vi "Powermeter_eom.vi"() -> ()   [LabVIEW 2016]
uses:
  <vilib>/userdefined/High Color/nirio_resource_hc.ctl
  <vilib>/FPGAPlugInAG/PXIe-7847R/niLvFpga_Open_PXIe-7847R.vi
  <vilib>/FPGAPlugInAG/PXIe-7847R/niLvFpga_Run_PXIe-7847R.vi
  <vilib>/Utility/error.llb/Error Cluster From Error Code.vi
  <vilib>/rvi/errors/niLvFpgaAdjustHostInterfaceError.vi
  <vilib>/Utility/file.llb/Write Delimited Spreadsheet (DBL).vi
  <vilib>/rvi/interface/nirviOpenFPGA/nirviOpenFPGA.xnode
  LabView Code/FPGA code/FPGA Bitfiles/Microspherefeedb_FPGATarget_MyCompilation_PIDXYZ_eom.lvbitx
  <vilib>/rvi/interface/nirviMethod/nirviMethod.xnode
  <vilib>/rvi/interface/nirviReadWriteControl/nirviReadWriteControl.xnode
  NiFpgaLv.dll
panel:
  in  "RIO Device":T1="RIO0"
  in  "N of steps":i32=401
  in  "step size":dbl=0.05
  in  "Start":dbl=-10.0
  in  "file path (dialog if empty)":path=path "C:/data/20180123/EOM_characterization/meas3.txt"
  out "Array":dbl[][](array[numeric])=[[0.000150393869, -10.0], [0.000149684973, -9.95], [0.000149058935, -9.9], [0.000148333784, -9.85], [0.000147686165, -9.8], [0.000147031693, -9.75], [0.0001463441, -9.7], [0.000145612459, -9.65], [0.000144846243, -9.6], [0.000144049729, -9.55], [0.000143292942, -9.5], [0.00014244036, -9.45], [0.000141621495, -9.4], [0.000140752702, -9.35], [0.000139932832, -9.3], [0.00013900231, -9.25], [0.000138039162, -9.2], [0.000137029376, -9.15], [0.000136068833, -9.1], [0.000135099486, -9.05], [0.000134103757, -9.0], [0.000133110167, -8.95], [0.000132204717, -8.9], [0.000131523033, -8.85], [0.000130512242, -8.8], [0.000129471417, -8.75], [0.000128434986, -8.7], [0.000127368286, -8.65], [0.00012630847, -8.6], [0.000125196137, -8.55], [0.00012410841, -8.5], [0.000123014004, -8.45], [0.000121917823, -8.4], [0.000120789067, -8.35], [0.000119675235, -8.3], [0.000118584379, -8.25], [0.00011747158, -8.2], [0.00011635691, -8.15], [0.00011528789, -8.1], [0.00011419248, -8.05], [0.000113120914, -8.0], [0.000112039837, -7.949999999999999], [0.000110946967, -7.9], [0.000109817694, -7.85], [0.000108703345, -7.8], [0.000107574131, -7.75], [0.000106449981, -7.699999999999999], [0.000105339168, -7.65], [0.000104231709, -7.6], [0.000103070852, -7.55], [0.000101967875, -7.5], [0.000100871737, -7.449999999999999], [9.97827883e-05, -7.4], [9.86708983e-05, -7.35], [9.75727817e-05, -7.3], [9.6466043e-05, -7.25], [9.53593917e-05, -7.199999999999999], [9.42729966e-05, -7.15], [9.31596442e-05, -7.1], [9.20545936e-05, -7.05], [9.0971429e-05, -7.0], [8.98795406e-05, -6.949999999999999], [8.87838905e-05, -6.9], [8.76979248e-05, -6.85], [8.66194823e-05, -6.8], [8.55211401e-05, -6.75], [8.44504029e-05, -6.699999999999999], [8.33811646e-05, -6.65], [8.23208466e-05, -6.6], [8.12596481e-05, -6.55], [8.02040886e-05, -6.5], [7.91571947e-05, -6.449999999999999], [7.80946066e-05, -6.4], [7.70534461e-05, -6.35], [7.60166076e-05, -6.3], [7.49777828e-05, -6.25], [7.39377138e-05, -6.199999999999999], [7.2927709e-05, -6.15], [7.19085219e-05, -6.1], [7.09057058e-05, -6.05], [6.99179145e-05, -6.0], [6.90001907e-05, -5.95], [6.81280071e-05, -5.8999999999999995], [6.72356837e-05, -5.85], [6.63338506e-05, -5.8], [6.53637835e-05, -5.75], [6.44089887e-05, -5.7], [6.34148528e-05, -5.6499999999999995], [6.24612585e-05, -5.6], [6.15193494e-05, -5.55], [6.05423993e-05, -5.5], [5.95535821e-05, -5.45], [5.8533682e-05, -5.3999999999999995], [5.7534915e-05, -5.35], [5.65688533e-05, -5.3], [5.5614415e-05, -5.25], [5.46966367e-05, -5.199999999999999], [5.37870292e-05, -5.1499999999999995], [5.28832607e-05, -5.1], [5.19945861e-05, -5.05], [5.11113103e-05, -5.0], [5.02308103e-05, -4.949999999999999], [4.93651132e-05, -4.8999999999999995], [4.85076816e-05, -4.85], [4.7653044e-05, -4.8], [4.6811776e-05, -4.75], [4.59838811e-05, -4.699999999999999], [4.51689448e-05, -4.6499999999999995], [4.43613535e-05, -4.6], [4.35506627e-05, -4.55], [4.27679734e-05, -4.5], [4.20016877e-05, -4.449999999999999], [4.12174413e-05, -4.3999999999999995], [4.04428574e-05, -4.35], [3.96582109e-05, -4.3], [3.88736553e-05, -4.25], [3.81013197e-05, -4.199999999999999], [3.73277762e-05, -4.1499999999999995], [3.65616252e-05, -4.1], [3.58079087e-05, -4.05], [3.50554728e-05, -4.0], [3.43142165e-05, -3.9499999999999993], [3.35744189e-05, -3.8999999999999995], [3.28419919e-05, -3.8499999999999996], [3.21193183e-05, -3.8], [3.14002464e-05, -3.75], [3.06878501e-05, -3.6999999999999993], [2.99921649e-05, -3.6499999999999995], [2.92990935e-05, -3.5999999999999996], [2.86223167e-05, -3.55], [2.79571123e-05, -3.5], [2.72917787e-05, -3.4499999999999993], [2.66343632e-05, -3.3999999999999995], [2.59851477e-05, -3.3499999999999996], [2.53385915e-05, -3.3], [2.46998134e-05, -3.25], [2.40559821e-05, -3.1999999999999993], [2.34006638e-05, -3.1499999999999995], [2.27987748e-05, -3.0999999999999996], [2.21989449e-05, -3.05], [2.1609243e-05, -3.0], [2.10390936e-05, -2.9499999999999993], [2.04805674e-05, -2.8999999999999995], [1.99267452e-05, -2.8499999999999996], [1.93897922e-05, -2.8], [1.8847466e-05, -2.75], [1.83229949e-05, -2.6999999999999993], [1.78147784e-05, -2.6499999999999995], [1.73084863e-05, -2.5999999999999996], [1.68125953e-05, -2.55], [1.63255063e-05, -2.5], [1.58559433e-05, -2.4499999999999993], [1.53885012e-05, -2.3999999999999995], [1.49266416e-05, -2.3499999999999996], [1.44811456e-05, -2.3], [1.40492502e-05, -2.25], [1.36235085e-05, -2.1999999999999993], [1.32113801e-05, -2.1499999999999995], [1.28091506e-05, -2.0999999999999996], [1.24163826e-05, -2.05], [1.20323566e-05, -2.0], [1.16541923e-05, -1.9499999999999993], [1.12883763e-05, -1.9000000000000004], [1.09351049e-05, -1.8499999999999996], [1.05901072e-05, -1.799999999999999], [1.02465801e-05, -1.75], [9.9213803e-06, -1.6999999999999993], [9.60321904e-06, -1.6500000000000004], [9.29292673e-06, -1.5999999999999996], [8.99726729e-06, -1.549999999999999], [8.70873282e-06, -1.5], [8.43643193e-06, -1.4499999999999993], [8.18091212e-06, -1.4000000000000004], [7.91727598e-06, -1.3499999999999996], [7.65832101e-06, -1.299999999999999], [7.40926771e-06, -1.25], [7.17645798e-06, -1.1999999999999993], [6.95599192e-06, -1.1500000000000004], [6.74318335e-06, -1.0999999999999996], [6.54176347e-06, -1.049999999999999], [6.3496891e-06, -1.0], [6.16568423e-06, -0.9499999999999993], [5.99233636e-06, -0.9000000000000004], [5.82761731e-06, -0.8499999999999996], [5.6737249e-06, -0.7999999999999989], [5.53044219e-06, -0.75], [5.39466873e-06, -0.6999999999999993], [5.26800886e-06, -0.6500000000000004], [5.1512161e-06, -0.5999999999999996], [5.04216541e-06, -0.5499999999999989], [4.94454116e-06, -0.5], [4.85808687e-06, -0.4499999999999993], [4.78006132e-06, -0.3999999999999986], [4.71090516e-06, -0.34999999999999964], [4.6509881e-06, -0.29999999999999893], [4.59980038e-06, -0.25], [4.56566067e-06, -0.1999999999999993], [4.53753364e-06, -0.14999999999999858], [4.51389815e-06, -0.09999999999999964], [4.50119205e-06, -0.049999999999998934], [4.49761546e-06, 0.0], [4.50493644e-06, 0.05000000000000071], [4.52040649e-06, 0.10000000000000142], [4.54338942e-06, 0.15000000000000036], [4.57284887e-06, 0.20000000000000107], [4.61270611e-06, 0.25], [4.66370693e-06, 0.3000000000000007], [4.72463398e-06, 0.3500000000000014], [4.79548862e-06, 0.40000000000000036], [4.87632133e-06, 0.45000000000000107], [4.96620123e-06, 0.5], [5.06512879e-06, 0.5500000000000007], [5.17437684e-06, 0.6000000000000014], [5.29454701e-06, 0.6500000000000004], [5.42475345e-06, 0.7000000000000011], [5.56434406e-06, 0.75], [5.71034434e-06, 0.8000000000000007], [5.86618762e-06, 0.8500000000000014], [6.03442004e-06, 0.9000000000000004], [6.22076232e-06, 0.9500000000000011], [6.40901635e-06, 1.0], [6.60227761e-06, 1.0500000000000007], [6.80729136e-06, 1.1000000000000014], [7.0222618e-06, 1.1500000000000004], [7.24339316e-06, 1.200000000000001], [7.47500917e-06, 1.25], [7.71556734e-06, 1.3000000000000007], [7.96448876e-06, 1.3500000000000014], [8.22485163e-06, 1.4000000000000004], [8.492304e-06, 1.450000000000001], [8.76691865e-06, 1.5], [9.05262095e-06, 1.5500000000000007], [9.34220316e-06, 1.6000000000000014], [9.64141054e-06, 1.6500000000000004], [9.94695256e-06, 1.700000000000001], [1.02618806e-05, 1.75], [1.05860536e-05, 1.8000000000000007], [1.09230805e-05, 1.8500000000000014], [1.12668922e-05, 1.9000000000000004], [1.16310439e-05, 1.950000000000001], [1.19824126e-05, 2.0], [1.23452683e-05, 2.0500000000000007], [1.27156709e-05, 2.1000000000000014], [1.31014122e-05, 2.1500000000000004], [1.3494483e-05, 2.200000000000001], [1.38967425e-05, 2.25], [1.4309092e-05, 2.3000000000000007], [1.47309238e-05, 2.3500000000000014], [1.51664326e-05, 2.4000000000000004], [1.5604548e-05, 2.450000000000001], [1.60573181e-05, 2.5], [1.65257334e-05, 2.5500000000000007], [1.70014682e-05, 2.6000000000000014], [1.7489805e-05, 2.6500000000000004], [1.79868839e-05, 2.700000000000001], [1.84921755e-05, 2.75], [1.90042283e-05, 2.8000000000000007], [1.9525809e-05, 2.8500000000000014], [2.00627619e-05, 2.9000000000000004], [2.06114837e-05, 2.950000000000001], [2.11680272e-05, 3.0], [2.1741831e-05, 3.0500000000000007], [2.23304087e-05, 3.1000000000000014], [2.29170873e-05, 3.1500000000000004], [2.35200441e-05, 3.200000000000001], [2.41231246e-05, 3.25], [2.47334319e-05, 3.3000000000000007], [2.53543731e-05, 3.3500000000000014], [2.59881981e-05, 3.4000000000000004], [2.66261377e-05, 3.450000000000001], [2.72773123e-05, 3.5], [2.79393644e-05, 3.5500000000000007], [2.86070172e-05, 3.6000000000000014], [2.92921013e-05, 3.6500000000000004], [2.99877356e-05, 3.700000000000001], [3.07035043e-05, 3.75], [3.14229328e-05, 3.8000000000000007], [3.21455518e-05, 3.8500000000000014], [3.28750029e-05, 3.9000000000000004], [3.35961195e-05, 3.950000000000001], [3.43051579e-05, 4.0], [3.50415103e-05, 4.050000000000001], [3.57838035e-05, 4.100000000000001], [3.65517044e-05, 4.15], [3.73171424e-05, 4.200000000000001], [3.80756319e-05, 4.25], [3.8799215e-05, 4.300000000000001], [3.95506904e-05, 4.350000000000001], [4.03167869e-05, 4.4], [4.11248147e-05, 4.450000000000001], [4.19666758e-05, 4.5], [4.28374588e-05, 4.550000000000001], [4.37859308e-05, 4.600000000000001], [4.47732164e-05, 4.65], [4.57099486e-05, 4.700000000000001], [4.66217934e-05, 4.75], [4.75081288e-05, 4.800000000000001], [4.84141528e-05, 4.850000000000001], [4.93323387e-05, 4.9], [5.02385046e-05, 4.950000000000001], [5.11602266e-05, 5.0], [5.20706235e-05, 5.050000000000001], [5.29692843e-05, 5.100000000000001], [5.39063658e-05, 5.15], [5.48410608e-05, 5.200000000000001], [5.57792373e-05, 5.25], [5.67410789e-05, 5.300000000000001], [5.77086103e-05, 5.350000000000001], [5.86976785e-05, 5.4], [5.96857863e-05, 5.450000000000001], [6.07094771e-05, 5.5], [6.17256883e-05, 5.550000000000001], [6.27655827e-05, 5.600000000000001], [6.383648e-05, 5.65], [6.48692512e-05, 5.700000000000001], [6.59068683e-05, 5.75], [6.6931214e-05, 5.800000000000001], [6.79607692e-05, 5.850000000000001], [6.8949681e-05, 5.9], [6.99779193e-05, 5.950000000000001], [7.09331798e-05, 6.0], [7.19119562e-05, 6.050000000000001], [7.27595689e-05, 6.100000000000001], [7.37930823e-05, 6.150000000000002], [7.48695602e-05, 6.199999999999999], [7.59697141e-05, 6.25], [7.7076118e-05, 6.300000000000001], [7.81868148e-05, 6.350000000000001], [7.93139698e-05, 6.400000000000002], [8.04390802e-05, 6.449999999999999], [8.1623024e-05, 6.5], [8.27808617e-05, 6.550000000000001], [8.40011926e-05, 6.600000000000001], [8.51979494e-05, 6.650000000000002], [8.6457243e-05, 6.699999999999999], [8.75623373e-05, 6.75], [8.87602946e-05, 6.800000000000001], [8.99671213e-05, 6.850000000000001], [9.11651732e-05, 6.900000000000002], [9.23712942e-05, 6.949999999999999], [9.36066863e-05, 7.0], [9.48174275e-05, 7.050000000000001], [9.60144171e-05, 7.100000000000001], [9.72127164e-05, 7.150000000000002], [9.84145154e-05, 7.199999999999999], [9.95925147e-05, 7.25], [0.000100772879, 7.300000000000001], [0.000101946309, 7.350000000000001], [0.000103158629, 7.400000000000002], [0.000104379353, 7.449999999999999], [0.000105610103, 7.5], [0.000106858803, 7.550000000000001], [0.000108113265, 7.600000000000001], [0.000109403249, 7.650000000000002], [0.000110698449, 7.699999999999999], [0.000111964153, 7.75], [0.000113197602, 7.800000000000001], [0.000114588809, 7.850000000000001], [0.000115792915, 7.900000000000002], [0.000117033196, 7.949999999999999], [0.000118301861, 8.0], [0.000119558063, 8.05], [0.000120717843, 8.100000000000001], [0.000121909376, 8.150000000000002], [0.000123119098, 8.2], [0.000124310172, 8.25], [0.000125538878, 8.3], [0.000126711224, 8.350000000000001], [0.000127905354, 8.400000000000002], [0.000129043823, 8.45], [0.00013023513, 8.5], [0.00013144796, 8.55], [0.000132647168, 8.600000000000001], [0.00013387794, 8.650000000000002], [0.000135094902, 8.7], [0.000136348492, 8.75], [0.00013752158, 8.8], [0.000138739255, 8.850000000000001], [0.000139946453, 8.900000000000002], [0.000141128767, 8.95], [0.000142247765, 9.0], [0.000143297293, 9.05], [0.000144258156, 9.100000000000001], [0.000145153375, 9.150000000000002], [0.000145910119, 9.200000000000003], [0.000146568229, 9.25], [0.000147048326, 9.3], [0.000147468018, 9.350000000000001], [0.000147810977, 9.400000000000002], [0.000148123741, 9.450000000000003], [0.000148378123, 9.5], [0.000148573919, 9.55], [0.000148743871, 9.600000000000001], [0.000148831081, 9.650000000000002], [0.000149022788, 9.700000000000003], [0.00014911592, 9.75], [0.000149254833, 9.8], [0.000149345811, 9.850000000000001], [0.000149377098, 9.900000000000002], [0.000149440675, 9.950000000000003], [0.000149476153, 10.0]]
  out "Power":dbl=0.000149476153
  in  "Wavelength (0.0)":dbl=1064.0
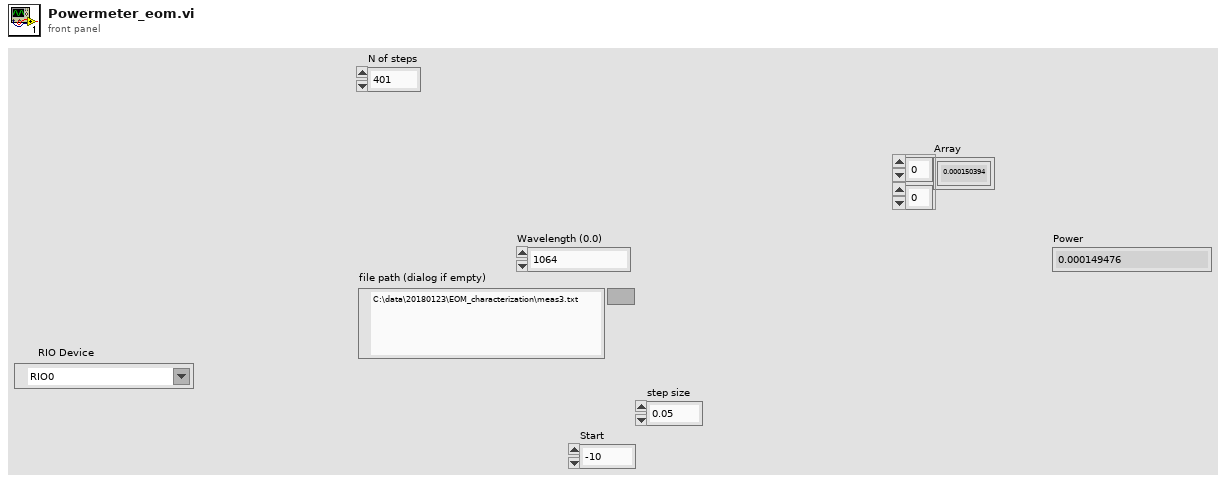
[diagram p1: front panel]
types:
  T1 = typedef "nirio_resource_hc.ctl" = tag
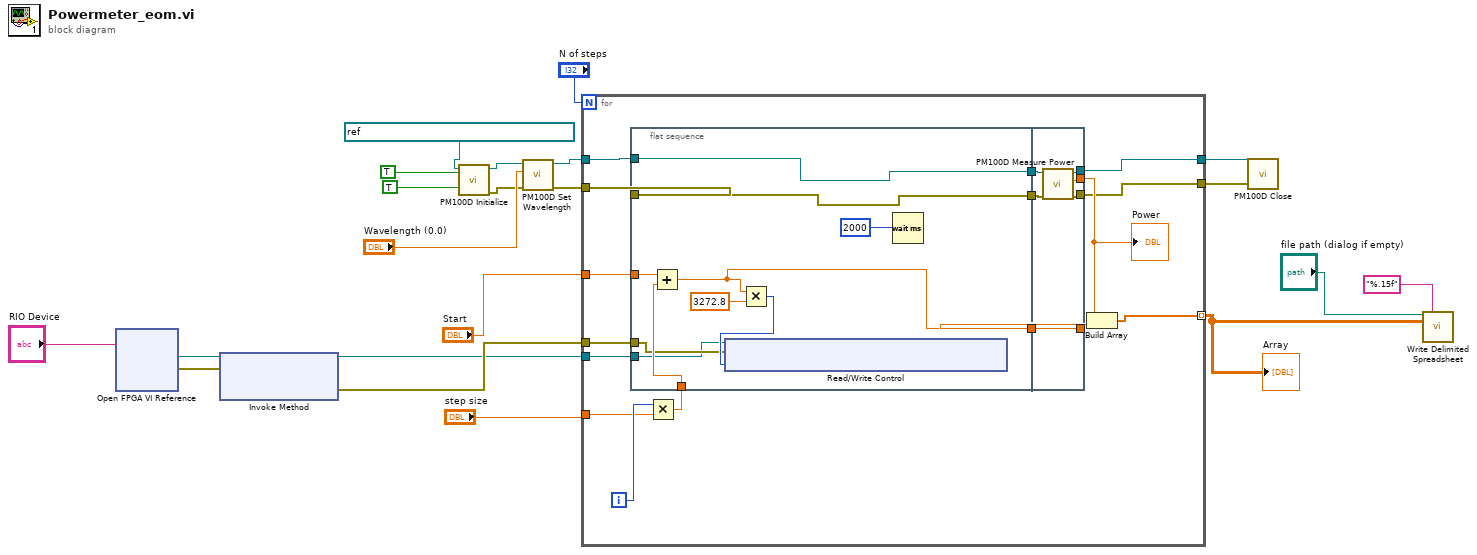
[diagram p0: block diagram]
diagram:
  n1 = xnode "Open FPGA VI Reference"("resource name"="RIO Device") -> ("FPGA VI Reference Out"=w4:refnum<k20>, "error out"=w3:errorcluster)  [unwired: 1 in]
  n2 = xnode "Invoke Method"("FPGA VI Reference In"=w4, "error in"=w3) -> ("FPGA VI Reference Out"=w1:refnum<k20>, "error out"=w2:errorcluster)  [unwired: 1 in]
  n3 = call <instrlib>:"PM100D Initialize.vi"("Reset Device (Reset Device)"=TRUE, "ID Query (Do Query)"=TRUE, "resource name"=refnum<visa-resource-name> "USB0::0x1313::0x8078::P0014456::INSTR") -> ("error out"=w15:errorcluster, "instrument handle out"=w17:refnum<visa-resource-name>)  [unwired: 7 in]
  n4 = call <instrlib>:"PM100D Set Wavelength.vi"("error in (no error)"=w15, "Wavelength (0.0)"="Wavelength (0.0)", "instrument handle"=w17) -> ("error out"=w14:errorcluster, "instrument handle out"=w16:refnum<visa-resource-name>)  [unwired: 7 in]
  n5 = for {
    N: "N of steps" -> [_]
    tunnel: "step size" -> [w36]
    tunnel: w16 -> [w33]
    tunnel: w14 -> [w32]
    tunnel: [w31] -> w13
    tunnel: [w30] -> w12
    tunnel: [w27] -> w11 mode=indexing
    tunnel: "Start" -> [w26]
    tunnel: w2 -> [w23]
    tunnel: w1 -> [w22]
    i -> [w37]
    n6 = flat-sequence {
      tunnel: w33 -> [w47]
      tunnel: w32 -> [w46]
      tunnel: [w47] -> w29
      tunnel: [w46] -> w28
      tunnel: w26 -> [w44]
      tunnel: w25 -> [w43]
      tunnel: [w42] -> w24
      tunnel: w23 -> [w39]
      tunnel: w22 -> [w38]
      tunnel: [w50] -> w30
      tunnel: [w49] -> w31
      tunnel: [w53] -> w34
      tunnel: [w48] -> w35
      tunnel: w29 -> [w52]
      tunnel: w28 -> [w51]
      tunnel: w24 -> [w53]
      frame #0 {
        n7 = Add(x=w44, y=w43) -> (x+y=w42:dbl)
        n8 = Multiply(x=w42, y=3272.8) -> (x*y=w40:i16)
        n9 = xnode "Read/Write Control"("FPGA VI Reference In"=w38, "error in"=w39, "EOM"=w40) -> ()  [unwired: 2 out]
        n10 = Wait (ms)(milliseconds to wait=u32 2000) -> ()  [unwired: 1 out]
      }
      frame #1 {
        n11 = call <instrlib>:"PM100D Measure Power.vi"("error in (no error)"=w51, "instrument handle"=w52) -> ("error out"=w50:errorcluster, "Power"=w48:dbl, "instrument handle out"=w49:refnum<visa-resource-name>)  [unwired: 7 in]
      }
    }
    n12 = Multiply(x=w37, y=w36) -> (x*y=w25:dbl)
    n13 = Build Array(w35, w34) -> (w27:dbl[])
    "Power" <- w35
  }
  "Array" <- w11
  n14 = call <instrlib>:"PM100D Close.vi"("error in (no error)"=w12, "instrument handle"=w13) -> ()  [unwired: 9 in, 1 out]
  n15 = call-poly <vilib>:"Write Delimited Spreadsheet.vi"("file path (dialog if empty)"="file path (dialog if empty)", "format (%.3f)"="%.15f", "2D data"=w11) -> ()  [unwired: 11 in, 2 out]
